vi "Criadir.vi"(0 "SOMENTE DIRETORIO":string) -> (1 "directory":bool, 2 "DIRETORIO":string)   [LabVIEW 2012]
doc: "Esta VI verifica se existe um diretorio no harddisk e se nao houver cria o respectivo diretorio."
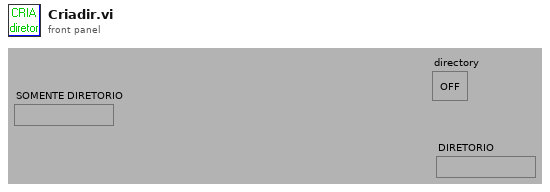
[diagram p1: front panel]
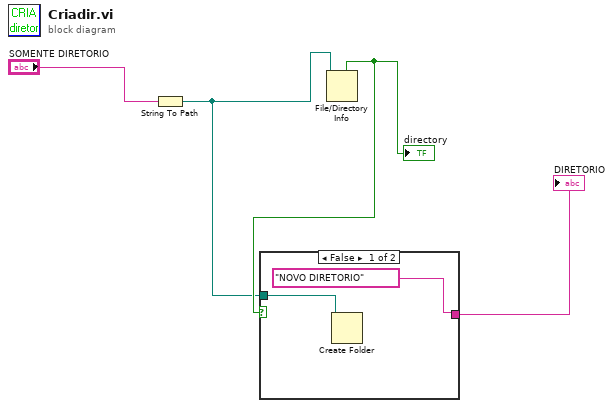
[diagram p0: block diagram]
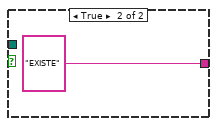
[diagram p2: hidden frame]
diagram:
  n1 = String To Path(string="SOMENTE DIRETORIO") -> (path=w2:path)
  n2 = File/Directory Info(path=w2) -> (directory=w3:bool)  [unwired: 1 in, 6 out]
  "directory" <- w3
  n3 = case shown="False" w3 {
    tunnel: ["NOVO DIRETORIO" "EXISTE"] -> w4
    tunnel: w2 -> [w6 _]
    frame False {
      n4 = Create Folder(path (use dialog)=w6) -> ()  [unwired: 2 in, 3 out]
    }
    frame True {
    }
  }
  "DIRETORIO" <- w4
